vi "ExSubGetSegCalib.vi"(0 "x dimension":u32, 1 "Pixel width":u32=25, 2 "Segment number":u32=1 min=1 step=1, 3 "error in (no error)":errorcluster, 4 "ini file":string) -> (5 "Calibrated Array":dbl[](array[numeric]) format="%.2f", 6 "Calibration Handle":u32, 7 "error out":errorcluster)   [LabVIEW 2010]
panel:
  # "ExSubGetSegCalib.vi : This sub vi is given a x \ndimension of ccd and pixel width and a segement\nnumber and ini file. It will read the ini file for\nthe segments calibration and generate a \ncalibrated array of x dimension."
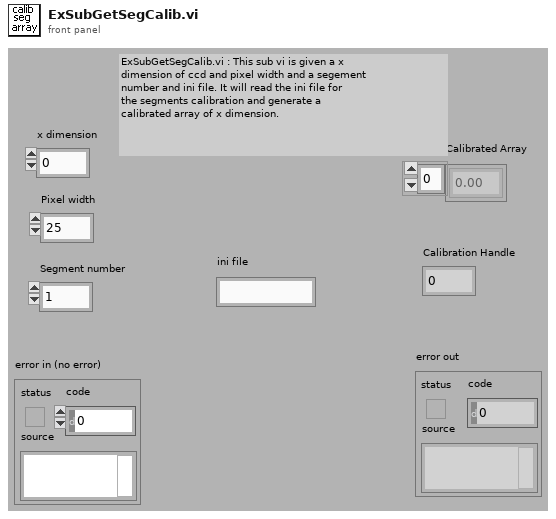
[diagram p1: front panel]
types:
  T1 = cluster{"Pixel width":u32, "Pixel width":u32, "x dimension":u32, i32, i32}
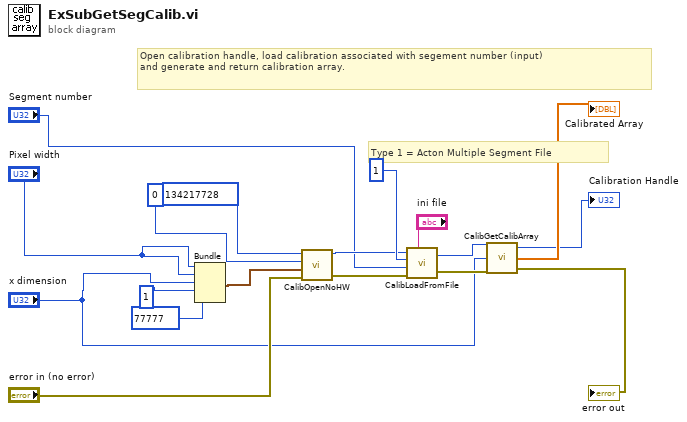
[diagram p0: block diagram]
diagram:
  # "Open calibration handle, load calibration associated with segement number (input)\nand generate and return calibration array."
  # "Type 1 = Acton Multiple Segment File"
  n1 = Bundle("Pixel width"="Pixel width", "Pixel width"="Pixel width", "x dimension"="x dimension", 1, 77777) -> (w13:T1)  [unwired: 1 in]
  n2 = call <userlib>:"CalibOpenNoHW.vi"("error in"="error in (no error)", "Data Info"=w13, "Calibration Type"=0, "Calibration Device ID"=134217728) -> ("error out"=w17:errorcluster, "Calibration Handle"=w16:u32)
  n3 = call <userlib>:"CalibLoadFromFile.vi"("File Path"="ini file", "error in (no error)"=w17, "Index"="Segment number", "File type"=1, "Calibration Handle"=w16) -> ("error out"=w10:errorcluster, "Calibration Handle"=w9:u32)  [unwired: 1 in]
  n4 = call <userlib>:"CalibGetCalibArray.vi"("error in"=w10, "Array Size"="x dimension", "Calibration Handle"=w9) -> ("error out"=→"error out":errorcluster, "Calibrated Array"=→"Calibrated Array":dbl[], "Calibration Handle"=→"Calibration Handle":u32)
